vi "GetMeasurements (1 GIPB).vi"() -> ()   [LabVIEW 2015]
uses:
  <vilib>/Utility/file.llb/Write Delimited Spreadsheet (DBL).vi
  <instrlib>/Keithley 2182/Keithley 2182.lvlib
panel:
  in  "DVM resource name":refnum<visa-resource-name>="GPIB0::17::INSTR"
  out "?":dbl=198.8220615594723
  in  "Current Set?":bool
  out "Manually Set Current":bool
  out "Complete?":bool
  in  "+B Field Added?":bool
  out "Ready To Change Field":bool
  in  "-B Field Added? 2":bool
  out "Ready To Change Field":bool
  in  "Voltage Measurement Path?":path=path "C:/Users/oodumosu/Desktop/KO StartUp/Test/ITO_Test0.txt"
  # "minutes"
  # "SetUp DVM"
  # "2:"
  # "1:"
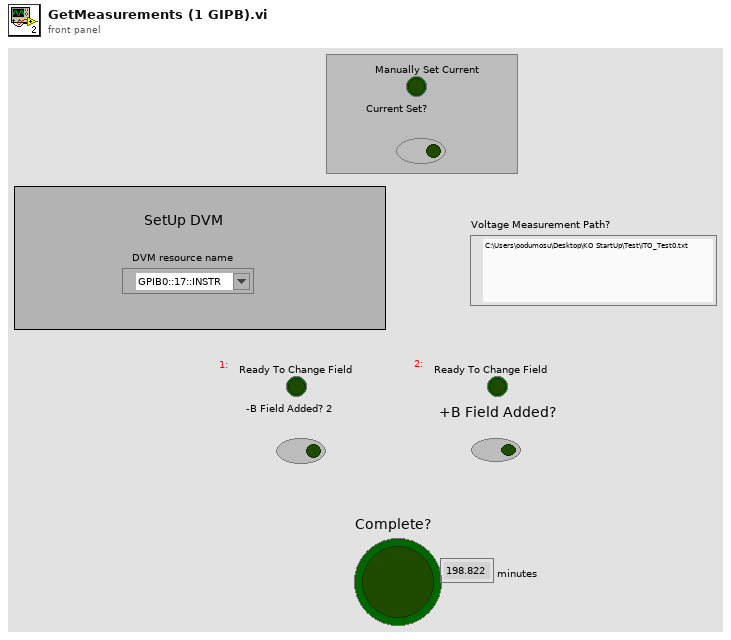
[diagram p1: front panel]
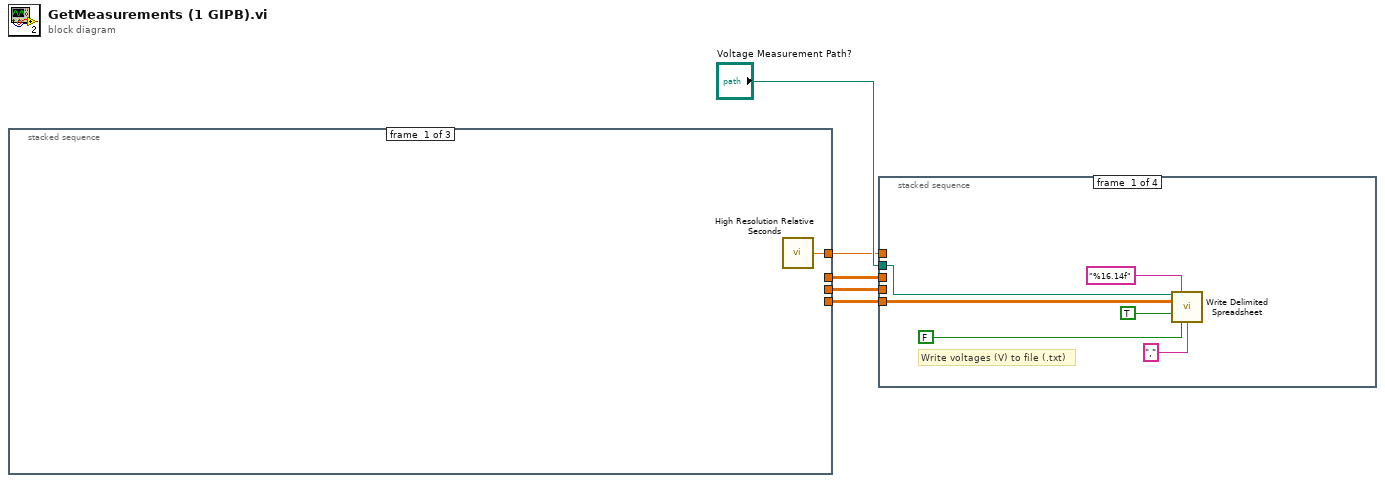
[diagram p0: block diagram]
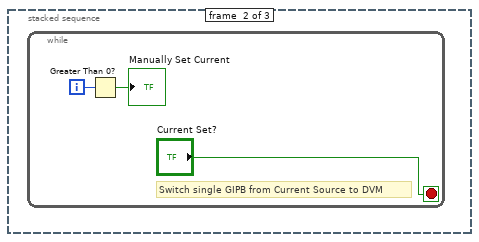
[diagram p2: hidden frame]
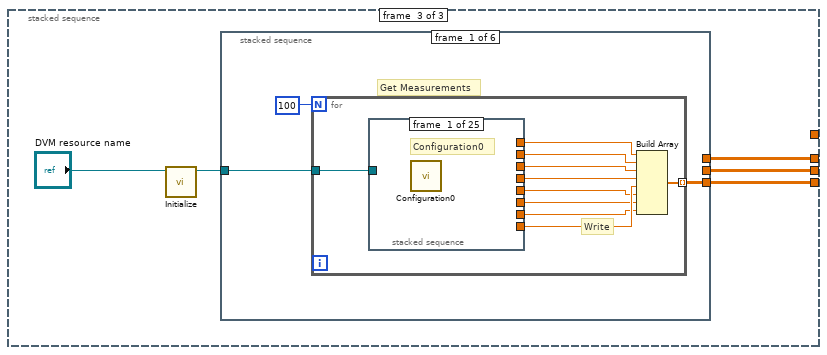
[diagram p3: hidden frame]
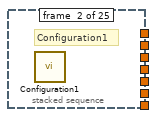
[diagram p4: hidden frame]
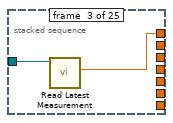
[diagram p5: hidden frame]
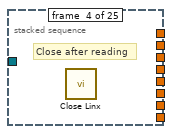
[diagram p6: hidden frame]
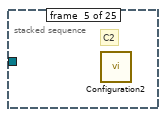
[diagram p7: hidden frame]
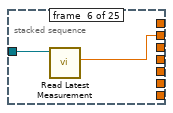
[diagram p8: hidden frame]
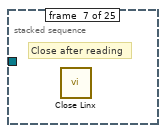
[diagram p9: hidden frame]
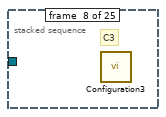
[diagram p10: hidden frame]
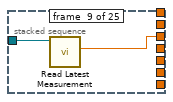
[diagram p11: hidden frame]
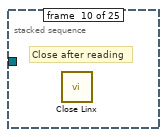
[diagram p12: hidden frame]
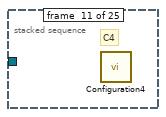
[diagram p13: hidden frame]
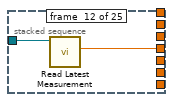
[diagram p14: hidden frame]
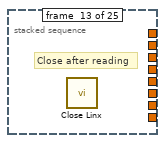
[diagram p15: hidden frame]
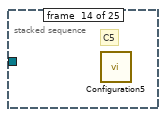
[diagram p16: hidden frame]
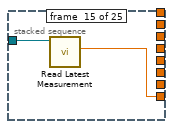
[diagram p17: hidden frame]
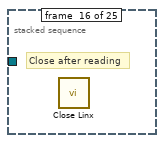
[diagram p18: hidden frame]
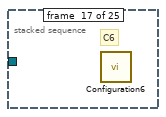
[diagram p19: hidden frame]
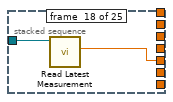
[diagram p20: hidden frame]
diagram:
  n1 = stacked-sequence {
    tunnel: [w6 _ _] -> w4
    tunnel: [_ _ w12] -> w3
    tunnel: [_ _ w11] -> w2
    tunnel: [_ _ w10] -> w1
    frame #0 {
      n2 = call <vilib>:"High Resolution Relative Seconds.vi"() -> ("relative seconds"=w6:dbl)
    }
    frame #1 {
      n3 = while {
        i -> [w8]
        stop <- "Current Set?" stop-if-true
        # "Switch single GIPB from Current Source to DVM"
        n4 = Greater Than 0?(x=w8) -> (x > 0?=→"Manually Set Current":bool)
      }
    }
    frame #2 {
      n5 = call <instrlib>:"Initialize.vi"("VISA resource name"="DVM resource name") -> ("VISA resource name out"=w13:refnum<visa-resource-name>)  [unwired: 9 in, 1 out]
      n6 = stacked-sequence {
        tunnel: [w16 _ _ _ _ _] -> w12
        tunnel: [_ _ w48 _ _ _] -> w11
        tunnel: [_ _ _ _ w69 _] -> w10
        tunnel: w13 -> [w15 _ w47 _ w67 _]
        frame #0 {
          # "Get Measurements"
          n7 = for {
            N: 100 -> [_]
            tunnel: [w27] -> w16 mode=indexing
            tunnel: w15 -> [w26]
            # "Write"
            n8 = stacked-sequence {
              tunnel: w26 -> [_ _ w29 _ _ w31 _ _ w33 _ _ w35 _ _ w37 _ _ w39 _ _ w41 _ _ w43 _]
              tunnel: [_ _ w28 _ _ _ _ _ _ _ _ _ _ _ _ _ _ _ _ _ _ _ _ _ _] -> w25
              tunnel: [_ _ _ _ _ w30 _ _ _ _ _ _ _ _ _ _ _ _ _ _ _ _ _ _ _] -> w24
              tunnel: [_ _ _ _ _ _ _ _ w32 _ _ _ _ _ _ _ _ _ _ _ _ _ _ _ _] -> w23
              tunnel: [_ _ _ _ _ _ _ _ _ _ _ w34 _ _ _ _ _ _ _ _ _ _ _ _ _] -> w22
              tunnel: [_ _ _ _ _ _ _ _ _ _ _ _ _ _ w36 _ _ _ _ _ _ _ _ _ _] -> w21
              tunnel: [_ _ _ _ _ _ _ _ _ _ _ _ _ _ _ _ _ w38 _ _ _ _ _ _ _] -> w20
              tunnel: [_ _ _ _ _ _ _ _ _ _ _ _ _ _ _ _ _ _ _ _ w40 _ _ _ _] -> w19
              tunnel: [_ _ _ _ _ _ _ _ _ _ _ _ _ _ _ _ _ _ _ _ _ _ _ w42 _] -> w18
              frame #0 {
                # "Configuration0"
                n9 = call "Configuration0.vi"() -> ()  [unwired: 12 in]
              }
              frame #1 {
                # "Configuration1"
                n10 = call "Configuration1.vi"() -> ()  [unwired: 12 in]
              }
              frame #2 {
                n11 = call <instrlib>:"Read Latest Measurement.vi"("VISA resource name"=w29) -> ("Measurement"=w28:dbl)  [unwired: 7 in, 3 out]
              }
              frame #3 {
                # "Close after reading"
                n12 = call "Close Linx.vi"() -> ()  [unwired: 12 in]
              }
              frame #4 {
                # "C2"
                n13 = call "Configuration2.vi"() -> ()  [unwired: 12 in]
              }
              frame #5 {
                n14 = call <instrlib>:"Read Latest Measurement.vi"("VISA resource name"=w31) -> ("Measurement"=w30:dbl)  [unwired: 7 in, 3 out]
              }
              frame #6 {
                # "Close after reading"
                n15 = call "Close Linx.vi"() -> ()  [unwired: 12 in]
              }
              frame #7 {
                # "C3"
                n16 = call "Configuration3.vi"() -> ()  [unwired: 12 in]
              }
              frame #8 {
                n17 = call <instrlib>:"Read Latest Measurement.vi"("VISA resource name"=w33) -> ("Measurement"=w32:dbl)  [unwired: 7 in, 3 out]
              }
              frame #9 {
                # "Close after reading"
                n18 = call "Close Linx.vi"() -> ()  [unwired: 12 in]
              }
              frame #10 {
                # "C4"
                n19 = call "Configuration4.vi"() -> ()  [unwired: 12 in]
              }
              frame #11 {
                n20 = call <instrlib>:"Read Latest Measurement.vi"("VISA resource name"=w35) -> ("Measurement"=w34:dbl)  [unwired: 7 in, 3 out]
              }
              frame #12 {
                # "Close after reading"
                n21 = call "Close Linx.vi"() -> ()  [unwired: 12 in]
              }
              frame #13 {
                # "C5"
                n22 = call "Configuration5.vi"() -> ()  [unwired: 12 in]
              }
              frame #14 {
                n23 = call <instrlib>:"Read Latest Measurement.vi"("VISA resource name"=w37) -> ("Measurement"=w36:dbl)  [unwired: 7 in, 3 out]
              }
              frame #15 {
                # "Close after reading"
                n24 = call "Close Linx.vi"() -> ()  [unwired: 12 in]
              }
              frame #16 {
                # "C6"
                n25 = call "Configuration6.vi"() -> ()  [unwired: 12 in]
              }
              frame #17 {
                n26 = call <instrlib>:"Read Latest Measurement.vi"("VISA resource name"=w39) -> ("Measurement"=w38:dbl)  [unwired: 7 in, 3 out]
              }
              frame #18 {
                # "Close after reading"
                n27 = call "Close Linx.vi"() -> ()  [unwired: 12 in]
              }
              frame #19 {
                # "C7"
                n28 = call "Configuration7.vi"() -> ()  [unwired: 12 in]
              }
              frame #20 {
                n29 = call <instrlib>:"Read Latest Measurement.vi"("VISA resource name"=w41) -> ("Measurement"=w40:dbl)  [unwired: 7 in, 3 out]
              }
              frame #21 {
                # "Close after reading"
                n30 = call "Close Linx.vi"() -> ()  [unwired: 12 in]
              }
              frame #22 {
                # "C8"
                n31 = call "Configuration8.vi"() -> ()  [unwired: 12 in]
              }
              frame #23 {
                n32 = call <instrlib>:"Read Latest Measurement.vi"("VISA resource name"=w43) -> ("Measurement"=w42:dbl)  [unwired: 7 in, 3 out]
              }
              frame #24 {
                # "Close after reading"
                n33 = call "Close Linx.vi"() -> ()  [unwired: 12 in]
              }
            }
            n34 = Build Array(w25, w24, w23, w22, w21, w20, w19, w18) -> (w27:dbl[])
          }
        }
        frame #1 {
          n35 = while {
            i -> [w45]
            stop <- "-B Field Added? 2" stop-if-true
            # "Add -B field"
            n36 = Greater Than 0?(x=w45) -> (x > 0?=→"Ready To Change Field":bool)
          }
        }
        frame #2 {
          n37 = for {
            N: 100 -> [_]
            tunnel: w47 -> [w55]
            tunnel: [w54] -> w48 mode=indexing
            n38 = stacked-sequence {
              tunnel: w55 -> [_ _ w57 _ _ w59 _ _ w61 _ _ w63 _]
              tunnel: [_ _ w56 _ _ _ _ _ _ _ _ _ _] -> w53
              tunnel: [_ _ _ _ _ w58 _ _ _ _ _ _ _] -> w52
              tunnel: [_ _ _ _ _ _ _ _ w60 _ _ _ _] -> w51
              tunnel: [_ _ _ _ _ _ _ _ _ _ _ w62 _] -> w50
              frame #0 {
                # "Reset"
                n39 = call "Configuration0.vi"() -> ()  [unwired: 12 in]
              }
              frame #1 {
                # "C9"
                n40 = call "Configuration9.vi"() -> ()  [unwired: 12 in]
              }
              frame #2 {
                n41 = call <instrlib>:"Read Latest Measurement.vi"("VISA resource name"=w57) -> ("Measurement"=w56:dbl)  [unwired: 7 in, 3 out]
              }
              frame #3 {
                # "Close after reading"
                n42 = call "Close Linx.vi"() -> ()  [unwired: 12 in]
              }
              frame #4 {
                # "C10"
                n43 = call "Configuration10.vi"() -> ()  [unwired: 12 in]
              }
              frame #5 {
                n44 = call <instrlib>:"Read Latest Measurement.vi"("VISA resource name"=w59) -> ("Measurement"=w58:dbl)  [unwired: 7 in, 3 out]
              }
              frame #6 {
                # "Close after reading"
                n45 = call "Close Linx.vi"() -> ()  [unwired: 12 in]
              }
              frame #7 {
                # "C11"
                n46 = call "Configuration11.vi"() -> ()  [unwired: 12 in]
              }
              frame #8 {
                n47 = call <instrlib>:"Read Latest Measurement.vi"("VISA resource name"=w61) -> ("Measurement"=w60:dbl)  [unwired: 7 in, 3 out]
              }
              frame #9 {
                # "Close after reading"
                n48 = call "Close Linx.vi"() -> ()  [unwired: 12 in]
              }
              frame #10 {
                # "C12"
                n49 = call "Configuration12.vi"() -> ()  [unwired: 12 in]
              }
              frame #11 {
                n50 = call <instrlib>:"Read Latest Measurement.vi"("VISA resource name"=w63) -> ("Measurement"=w62:dbl)  [unwired: 7 in, 3 out]
              }
              frame #12 {
                # "Close after reading"
                n51 = call "Close Linx.vi"() -> ()  [unwired: 12 in]
              }
            }
            n52 = Build Array(w53, w52, w51, w50) -> (w54:dbl[])
          }
        }
        frame #3 {
          # "Change to +B Field"
          n53 = while {
            i -> [w64]
            stop <- "+B Field Added?" stop-if-true
            n54 = Greater Than 0?(x=w64) -> (x > 0?=→"Ready To Change Field":bool)
          }
        }
        frame #4 {
          n55 = for {
            N: 100 -> [_]
            tunnel: w67 -> [w75]
            tunnel: [w70] -> w69 mode=indexing
            n56 = stacked-sequence {
              tunnel: w75 -> [_ _ w77 _ _ w79 _ _ w81 _ _ w83 _]
              tunnel: [_ _ w76 _ _ _ _ _ _ _ _ _ _] -> w74
              tunnel: [_ _ _ _ _ w78 _ _ _ _ _ _ _] -> w73
              tunnel: [_ _ _ _ _ _ _ _ w80 _ _ _ _] -> w72
              tunnel: [_ _ _ _ _ _ _ _ _ _ _ w82 _] -> w71
              frame #0 {
                # "Reset"
                n57 = call "Configuration0.vi"() -> ()  [unwired: 12 in]
              }
              frame #1 {
                # "C13"
                n58 = call "Configuration9.vi"() -> ()  [unwired: 12 in]
              }
              frame #2 {
                n59 = call <instrlib>:"Read Latest Measurement.vi"("VISA resource name"=w77) -> ("Measurement"=w76:dbl)  [unwired: 7 in, 3 out]
              }
              frame #3 {
                # "Close after reading"
                n60 = call "Close Linx.vi"() -> ()  [unwired: 12 in]
              }
              frame #4 {
                # "C14"
                n61 = call "Configuration10.vi"() -> ()  [unwired: 12 in]
              }
              frame #5 {
                n62 = call <instrlib>:"Read Latest Measurement.vi"("VISA resource name"=w79) -> ("Measurement"=w78:dbl)  [unwired: 7 in, 3 out]
              }
              frame #6 {
                # "Close after reading"
                n63 = call "Close Linx.vi"() -> ()  [unwired: 12 in]
              }
              frame #7 {
                # "C15"
                n64 = call "Configuration11.vi"() -> ()  [unwired: 12 in]
              }
              frame #8 {
                n65 = call <instrlib>:"Read Latest Measurement.vi"("VISA resource name"=w81) -> ("Measurement"=w80:dbl)  [unwired: 7 in, 3 out]
              }
              frame #9 {
                # "Close after reading"
                n66 = call "Close Linx.vi"() -> ()  [unwired: 12 in]
              }
              frame #10 {
                # "C16"
                n67 = call "Configuration12.vi"() -> ()  [unwired: 12 in]
              }
              frame #11 {
                n68 = call <instrlib>:"Read Latest Measurement.vi"("VISA resource name"=w83) -> ("Measurement"=w82:dbl)  [unwired: 7 in, 3 out]
              }
              frame #12 {
                # "Close after reading"
                n69 = call "Close Linx.vi"() -> ()  [unwired: 12 in]
              }
            }
            n70 = Build Array(w74, w73, w72, w71) -> (w70:dbl[])
          }
        }
        frame #5 {
          "Complete?" <- TRUE
        }
      }
    }
  }
  n71 = stacked-sequence {
    tunnel: "Voltage Measurement Path?" -> [w86 w92 w98 _]
    tunnel: w3 -> [w85 _ _ _]
    tunnel: w2 -> [_ w91 _ _]
    tunnel: w4 -> [_ _ _ w103]
    tunnel: w1 -> [_ _ w97 _]
    frame #0 {
      # "Write voltages (V) to file (.txt)"
      n72 = call-poly <vilib>:"Write Delimited Spreadsheet.vi"("file path (dialog if empty)"=w86, "format (%.3f)"="%16.14f", "2D data"=w85, "append to file? (F)"=TRUE, "transpose? (F)"=FALSE, "delimiter (\\t)"="," ("delimiter (\\t)")) -> ()  [unwired: 8 in, 2 out]
    }
    frame #1 {
      # "Write voltages (V) to file (.txt)"
      n73 = call-poly <vilib>:"Write Delimited Spreadsheet.vi"("file path (dialog if empty)"=w92, "format (%.3f)"="%16.14f", "2D data"=w91, "append to file? (F)"=TRUE, "transpose? (F)"=FALSE, "delimiter (\\t)"="," ("delimiter (\\t)")) -> ()  [unwired: 8 in, 2 out]
    }
    frame #2 {
      n74 = call-poly <vilib>:"Write Delimited Spreadsheet.vi"("file path (dialog if empty)"=w98, "format (%.3f)"="%16.14f", "2D data"=w97, "append to file? (F)"=TRUE, "transpose? (F)"=FALSE, "delimiter (\\t)"="," ("delimiter (\\t)")) -> ()  [unwired: 8 in, 2 out]
    }
    frame #3 {
      # "Calculate and display total run time of program"
      n75 = call <vilib>:"High Resolution Relative Seconds.vi"() -> ("relative seconds"=w107:dbl)
      n76 = Subtract(x=w107, y=w103) -> (x-y=w106:dbl)
      n77 = Divide(x=w106, y=60.0) -> (x/y=→"?":dbl)
    }
  }
